vi "AlliGator Current Time Point.vi"(8 "Error In":errorcluster, 9 "Current Dataset Path":path, 10 "Time-Series Paths":path[](array[path]), 11 "Time Series Timestamps":dbl[](array[numeric])) -> (0 "Error Out":errorcluster, 2 "Time Point":i32, 3 "Current Time Stamp":dbl)   [LabVIEW 2021, in "AlliGator Files.lvlib"]
doc: "Returns the current dataset's timestamp, either from the stored array of timestamp or if it is empty, from the \"Current Frame Timestamp\" internal variable."
uses:
  AlliGator Files.lvlib
  AlliGator Variables List.ctl
  Variant/Variant to Data/Variant to DBL.vi
  AlliGator Globals, Variables & Constants.lvlib
  Variant/Variant to Data/Variant to Data.lvlib
panel:
  # "see the AlliGator License on the block diagram (Ctrl+E or Window:Show Block Diagram)"
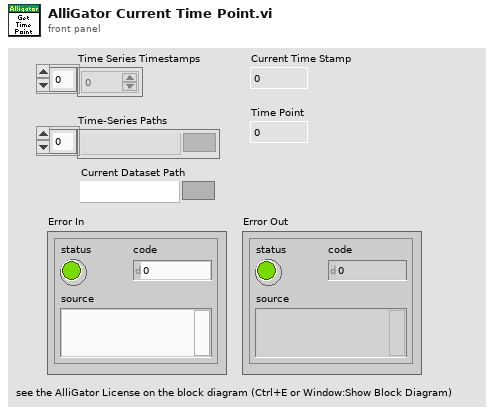
[diagram p1: front panel]
types:
  T1 = typedef "AlliGator Globals, Variables & Constants.lvlib/AlliGator Variables List.ctl" = enum16{"---- GUI ----", "GUI:Initialization Status", "GUI:State Indicators Refnum", "GUI:Original AlliGator Menu Items", "GUI:Current Action Loop State", "GUI:Script in progress", "GUI:Playback", "GUI:Loop Playback", "GUI:Search ROI Used", "GUI:Search ROI", "Decay Graph Max Legend Size", "Intensity Graph Max Legend Size", "Decay Statistics Graph Max Legend Size", "Phasor Graph Max Legend Size", "Phasor Ratio Graph Max Legend Size", "Lifetime Graph Max Legend Size", "---- Files ----", "Files:Export Dataset Frames as Individual Files", "Files:Show Batch Export Help Balloons", "Files:Frames in Dataset", "Files:ptu File Frame Start Indices", "Files:Current Frame in Dataset", "Files:Current Frame Timestamp", "Files:Dataset Loaded", "Files:Dataset Metadata", "Files:Dataset Channel", "Files:Dataset Data Description", "Files:Background Dataset Metadata", "Files:Background Dataset Channel", "Files:Background Dataset Data Description", "Files:Background File Subtraction", "Files:Background File Path", "Files:Background File Pile-up Correction", "Files:Background File Pixel Well Capacity", "Files:Background File Scaling Factor", "Files:Current Dataset Load Settings", "Files:Dataset Path", "------ Python Plugins ------", "Python Plugins:Information", "Python Plugins:Python Session", "Python Plugins:Valid Python Session?", "---- Source Image ----", "Source Image:ROIs", "Source Image:Current ROI", "Source Image ROI Event Refnum", "X_Source Image Display Range", "X_Source Image Palette Information", "Source Image:Palette List", "Source Image:Scale", "Source Image:ROI Overlay Color", "Source Image:ICCD-specific Information", "---- Image Profile Window ----", "Image Profile:Overlay ROI in Source Image", "Image Profile Window Event Refnum", "Image Profile:IntensityType", "Image Profile:Intensity Average Type", "Image Profile:Intensity-weighted SDV", "Image Profile:Box Profile Type", "Image Profile Window Open", "Image Profile:Plotted Fit Parameter", "X_Type of Displayed Image", "X_Time Gate Slider", "Source Image:Overlay to Erase", "Is Displayed Image Accumulated", "White Light Image Modified", "Mask Image Modified", "Macrotime Gate Separation", "------ Phasor Graph -------", "Phasor Graph:Show Line", "---- Phasor Plot ---", "Phasor Plot Parameters Changed", "FLI Dataset Modified since last Phasor Plot Calculation", "Phasor Harmonics Data", "Selected Phasor Harmonics", "Phasor Harmonic Manager Event Refnum", "Phasor Plot ROIs", "Current Phasor Plot ROI", "Phasor Plot ROI Event Refnum", "Phasor Plot Image Reference Points", "Phasor Plot Computed", "Phasor Plot Palette Information", "Phasor Plot Palette List", "Phasor Ratio Palette Information", "Phasor Ratio Palette List", "Phasor Image Scale", "Phasor Plot Image Overlay to Erase", "Phasor Plot Image Elements to Update", "Current Phasor Plot Calculation Parameters", "Current Phasor Calibration Options", "Reset Cumulated Phasor Plot", "Phasor Ratio Reference 1", "Phasor Ratio Lifetime Reference 1", "Phasor Ratio Reference 1 Frequency", "Phasor Ratio Reference 2", "Phasor Ratio Lifetime Reference 2", "Phasor Ratio Reference 2 Frequency", "---- Decay Analysis ----", "Number of Selected Decays to Fit", "LS Fit Results", "LAR Fit Results", "BS Fit Results", "Last Decay Max - Min", "Best Fit Parameters", "Best Fit Parameter Names", "Actual Size X", "Actual Size Y", "Binning X", "Binning Y", "Actual # Gates", "Dataset Number", "Gates to...", "Gates Skipped", "Gates to keep", "Gate Step", "Gate Separation", "Reversed Gates", "Pile-up Correction", "Pixel Well Capacity", "Background Subtracted", "Background Subtraction Method", "Background Definition Range", "Background File (deprecated)", "Number of Dataset Accumulated", "Array of Accumulated Dataset Paths", "Do Averaged Datasets", "Destination File Path", "Process Plot Target", "Use 1/D as Phasor Frequency", "---- Decay Fit Parameter Map -----", "Decay Fit Parameter Map Palette Information", "Decay Fit Parameter Map Palette List", "Local Decay Graph Window Event Refnum", "------- Local Decay Window ---------", "Use normalized IRF for convolution", "----- Miscellaneous ----", "Skippable Dialog Windows Status"}
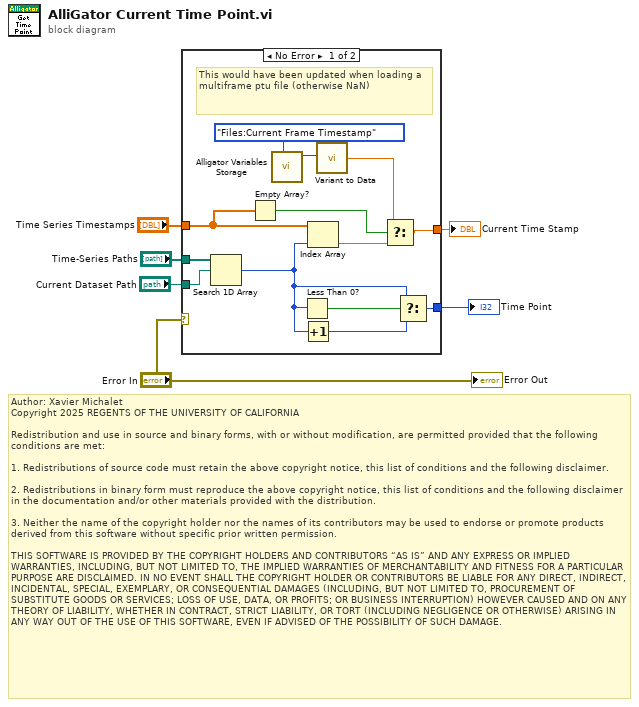
[diagram p0: block diagram]
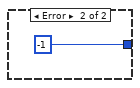
[diagram p2: hidden frame]
diagram:
  # "Author: Xavier Michalet\nCopyright 2025 REGENTS OF THE UNIVERSITY OF CALIFORNIA\n\nRedistribution and use in source and binary forms, with or without modification, are permitted provided that the following conditions are met:\n\n1. Redistributions of source code must retain the above copyright notice, this list of conditions and the following disclaimer.\n\n2. Redistributions in binary form must reproduce the above copyright notice, this list of conditions and the following disclaimer in the documentation and/or other materials provided with the distribution.\n\n3. Neither the name of the copyright holder nor the names of its contributors may be used to endorse or promote products derived from this software without specific prior written permission.\n\nTHIS SOFTWARE IS PROVIDED BY THE COPYRIGHT HOLDERS AND CONTRIBUTORS “AS IS” AND ANY EXPRESS OR IMPLIED WARRANTIES, INCLUDING, BUT NOT LIMITED TO, THE IMPLIED WARRANTIES OF MERCHANTABILITY AND FITNESS FOR A PARTICULAR PURPOSE ARE DISCLAIMED. IN NO EVENT SHALL THE COPYRIGHT HOLDER OR CONTRIBUTORS BE LIABLE FOR ANY DIRECT, INDIRECT, INCIDENTAL, SPECIAL, EXEMPLARY, OR CONSEQUENTIAL DAMAGES (INCLUDING, BUT NOT LIMITED TO, PROCUREMENT OF SUBSTITUTE GOODS OR SERVICES; LOSS OF USE, DATA, OR PROFITS; OR BUSINESS INTERRUPTION) HOWEVER CAUSED AND ON ANY THEORY OF LIABILITY, WHETHER IN CONTRACT, STRICT LIABILITY, OR TORT (INCLUDING NEGLIGENCE OR OTHERWISE) ARISING IN ANY WAY OUT OF THE USE OF THIS SOFTWARE, EVEN IF ADVISED OF THE POSSIBILITY OF SUCH DAMAGE."
  n1 = case shown="No Error" "Error In" {
    tunnel: "Time-Series Paths" -> [w19 _]
    tunnel: "Current Dataset Path" -> [w18 _]
    tunnel: "Time Series Timestamps" -> [w13 _]
    tunnel: [w10 _] -> w3
    tunnel: [w14 -1 ("index of element")] -> w2
    frame No Error {
      # "This would have been updated when loading a multiframe ptu file (otherwise NaN)"
      n2 = Search 1D Array(1D array=w19, element=w18) -> (index of element=w16:i32)  [unwired: 1 in]
      n3 = Empty Array?(array=w13) -> (empty?=w11:bool)
      n4 = call "Alligator Variables Storage.vi"("AlliGator Variable"=AlliGator_Variables_List."Files:Current Frame Timestamp" ("Alligator Variable")) -> ("Data out"=w8:variant)  [unwired: 8 in, 2 out]
      n5 = Less Than 0?(x=w16) -> (x < 0?=w17:bool)
      n6 = Increment(x=w16) -> (x+1=w15:i32)
      n7 = Index Array(array=w13, index=w16) -> (element=w12:dbl)
      n8 = call-poly "Variant to Data.vi"("Variant"=w8) -> ("Value"=w7:dbl)  [unwired: 8 in]
      n9 = Select(t=w7, s=w11, f=w12) -> (s? t:f=w10:dbl)
      n10 = Select(t=w16, s=w17, f=w15) -> (s? t:f=w14:i32)
    }
    frame Error {
    }
  }
  "Time Point" <- w2
  "Current Time Stamp" <- w3
  "Error Out" <- "Error In"
